vi "calibrationSpectrometer_getEvent_Heartbeat.vi"(8 "error in (no error)":errorcluster, 11 "logevent_Heartbeat_Ctl":T1) -> (0 "error out":errorcluster, 2 "function return":i32, 3 "logevent_Heartbeat_Ctl out":T1)   [LabVIEW 2016, in "SALLV_calibrationSpectrometer.lvlib"]
doc: "int calibrationSpectrometer_shm_getEvent_HeartbeatLV(calibrationSpectrometer_logevent_HeartbeatLV *logevent_Heartbeat_Ctl );"
uses:
  SALLV_calibrationSpectrometer.lvlib
  DataTypes/logevent_Heartbeat.ctl
  SALLV_calibrationSpectrometer.so
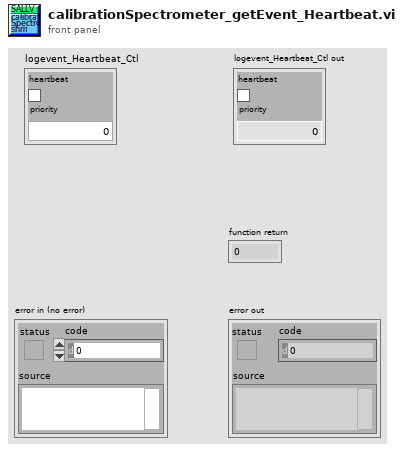
[diagram p1: front panel]
types:
  T1 = typedef "SALLV_calibrationSpectrometer.lvlib/logevent_Heartbeat.ctl" = cluster{"heartbeat":bool, "priority":i32}
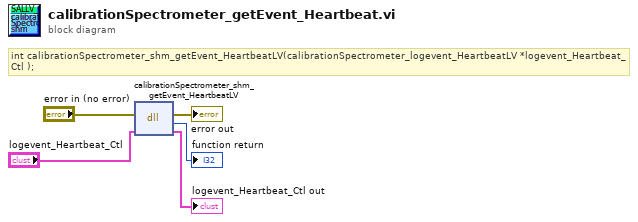
[diagram p0: block diagram]
diagram:
  # "int calibrationSpectrometer_shm_getEvent_HeartbeatLV(calibrationSpectrometer_logevent_HeartbeatLV *logevent_Heartbeat_Ctl );"
  n1 = dll-call lib="home/harini/TCS/sallv_sedspectrometer/SALLV_calibrationSpectrometer.*" fn="calibrationSpectrometer_shm_getEvent_HeartbeatLV"(error in="error in (no error)", "logevent_Heartbeat_Ctl"="logevent_Heartbeat_Ctl") -> (error out=→"error out":errorcluster, →"function return":i32, "logevent_Heartbeat_Ctl"=→"logevent_Heartbeat_Ctl out":T1)  [unwired: 2 in, 1 out]
